vi "ModbusRdWrStatus.vi"() -> ()   [LabVIEW 2020]
uses:
  <vilib>/Modbus/master/Create Master Instance (TCP).vi
  <vilib>/Modbus/master/Modbus Master.lvclass
panel:
  out "Error":bool
  in  "ip":string="192.168.0.50"
  out "Timer":u16
  in  "Servo 5":i16=6
  in  "Servo 4":i16=5
  in  "Servo 3":i16=4
  in  "Servo 2":i16=3
  in  "Servo 1":i16=2
  in  "Servo 0":i16=1
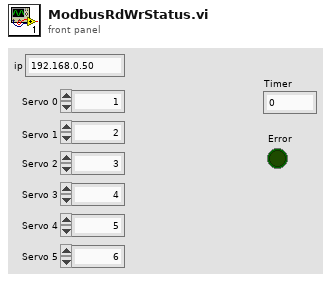
[diagram p1: front panel]
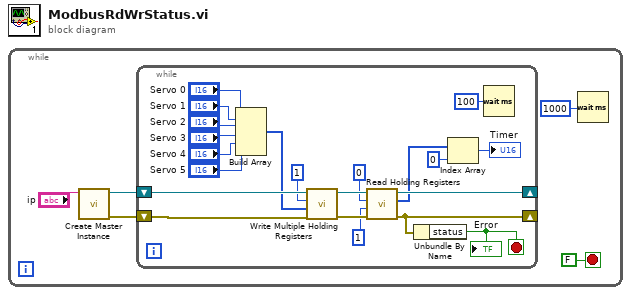
[diagram p0: block diagram]
diagram:
  n1 = while {
    stop <- FALSE stop-if-true
    n2 = call-poly <vilib>:"Create Master Instance.vi"("address"="ip") -> ("error out"=w3:errorcluster, "TCP master instance"=w4:refnum<class "Modbus Master.lvclass">)  [unwired: 9 in]
    n3 = while {
      shift-right: [w14] -> _
      shift-left: w4 -> [w20]
      shift-right: [w7] -> _
      shift-left: w3 -> [w8]
      stop <- w6 stop-if-true
      n4 = Build Array("Servo 0", "Servo 1", "Servo 2", "Servo 3", "Servo 4", "Servo 5") -> (w19:i16[])
      n5 = call-dynamic "Write Multiple Holding Registers.vi"("error in (no error)"=w8, "holding register values"=w19, "starting address"=u16 1, "Modbus master in"=w20) -> ("error out"=w13:errorcluster, "Modbus master out"=w15:refnum<class "Modbus Master.lvclass">)  [unwired: 6 in]
      n6 = call-dynamic "Read Holding Registers.vi"("error in (no error)"=w13, "number of holding registers"=u16 1, "starting address"=u16 0, "Modbus master in"=w15) -> ("error out"=w7:errorcluster, "register values"=w10:u16[], "Modbus master out"=w14:refnum<class "Modbus Master.lvclass">)  [unwired: 5 in]
      n7 = Unbundle By Name(w7) -> ("status"=w6:bool)
      "Error" <- w6
      n8 = Index Array(array=w10, index=0) -> (element=→"Timer":u16)
      n9 = Wait (ms)(milliseconds to wait=u32 100) -> ()  [unwired: 1 out]
    }
    n10 = Wait (ms)(milliseconds to wait=1000) -> ()  [unwired: 1 out]
  }
